vi "DialogTF.vi"(8 "error in (no error)":errorcluster, 9 "F button name (\"Cancel\")":string, 10 "T button name (\"OK\")":string, 11 "message":string) -> (0 "error out":errorcluster, 2 "T button?":bool)   [LabVIEW 2014]
panel:
  # "LICENSED MATERIALS – PROPERTY OF IBM\nCopyright IBM Corp. 2016,\nALL RIGHTS RESERVED"
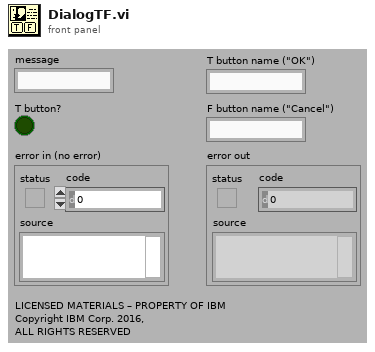
[diagram p1: front panel]
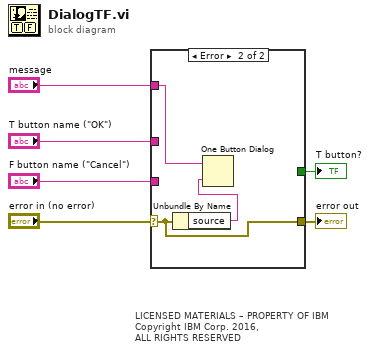
[diagram p0: block diagram]
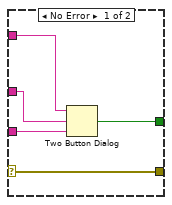
[diagram p2: hidden frame]
diagram:
  # "LICENSED MATERIALS – PROPERTY OF IBM\nCopyright IBM Corp. 2016,\nALL RIGHTS RESERVED"
  n1 = case shown="Error" "error in (no error)" {
    selector: "error in (no error)" -> [w11 w14]
    tunnel: "message" -> [w10 w13]
    tunnel: [w11 w14] -> w5
    tunnel: "T button name (\"OK\")" -> [w9 _]
    tunnel: "F button name (\"Cancel\")" -> [w8 _]
    tunnel: [w7 _] -> w1
    frame No Error {
      n2 = Two Button Dialog(message=w10, 1:w8, 2:w9) -> (T button?=w7:bool)
    }
    frame Error {
      n3 = Unbundle By Name(w14) -> ("source"=w12:string)
      n4 = One Button Dialog(message=w13, button name ("OK")=w12) -> ()  [unwired: 1 out]
    }
  }
  "error out" <- w5
  "T button?" <- w1
